vi "WPI_CompressorStart.vi"(8 "error in (no error)":errorcluster, 11 "CompressorDevRef":T1) -> (0 "error out":errorcluster, 3 "CompressorDevRef":T1)   [LabVIEW 2017]
doc: "Starts the monitoring and updating of the compressor. Use the Open VI to open a reference to the compressor before you use this VI.\n\nThis software is licensed. Open the labview\\readme\\WPI Robotics Library Open Source License.txt file for more information."
uses:
  <vilib>/Rock Robotics/WPI/Compressor/WPI_CompressorDevRef.ctl
  <vilib>/Rock Robotics/WPI/CAN/PCM/WPI_CAN_PCMGlobalOps.ctl
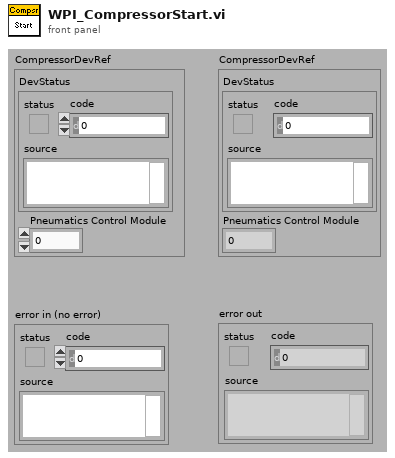
[diagram p1: front panel]
types:
  T1 = typedef "WPI_CompressorDevRef.ctl" = cluster{"DevStatus":errorcluster, "Pneumatics Control Module":u8}
  T2 = typedef "WPI_CAN_PCMGlobalOps.ctl" = enum16{"Read For Send", "Write After Receive", "Set Solenoids", "Set Closed Loop", "Clear Sticky Faults", "Get All", "Write Error", "Write After Receive Blacklist", "Set Control Frame Rate"}
  T3 = cluster{"Solenoid Status":bool[], "Battery Voltage":dbl, "Solenoid Voltage":dbl, "Compressor Current":dbl, "CompressorEnabled":bool, "StickySolenoidFault":bool, "StickyCompressorFault":bool, "SolenoidFault":bool, "CompressorFault":bool, "HardwareFault":bool, "ClosedLoopStatus":bool, "PressureStatus":bool, "Module Enabled":bool, "ClosedLoopSuggestedOutput":bool, "CAN Error":errorcluster, "Sticky Solenoid Faults":bool[]}
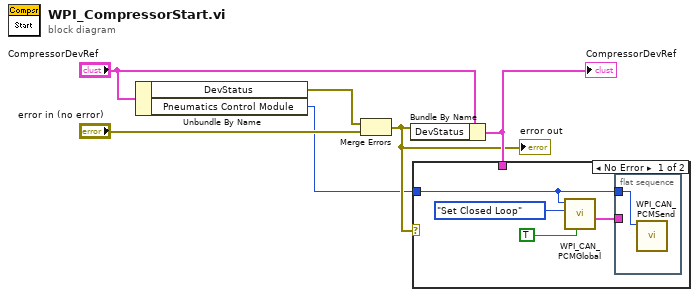
[diagram p0: block diagram]
diagram:
  n1 = Unbundle By Name("CompressorDevRef") -> ("DevStatus"=w4:errorcluster, "Pneumatics Control Module"=w1:u8)
  n2 = Merge Errors(w4, "error in (no error)") -> (w2:errorcluster)
  "error out" <- w2
  n3 = Bundle By Name(cluster="CompressorDevRef", "DevStatus"=w2) -> (w3:T1)
  "CompressorDevRef" <- w3
  n4 = case shown="No Error" w2 {
    tunnel: w3 -> [_ _]
    tunnel: w1 -> [w8 _]
    frame No Error {
      n5 = call <vilib>:"WPI_CAN_PCMGlobal.vi"("Set Value"=TRUE (".not. x?"), "Operation"=WPI_CAN_PCMGlobalOps."Set Closed Loop", "Pneumatics Control Module (0)"=w8) -> ("Get All"=w9:T3)  [unwired: 6 in, 2 out]
      n6 = flat-sequence {
        tunnel: w9 -> [_]
        tunnel: w8 -> [w11]
        frame #0 {
          n7 = call <vilib>:"WPI_CAN_PCMSend.vi"("Pneumatics Control Module (0)"=w11) -> ()  [unwired: 10 in, 1 out]
        }
      }
    }
    frame Error {
    }
  }
